vi "Data Viewer.vi"(8 "error in (no error)":errorcluster, 10 "Starting Waveforms":waveform(dbl)[](array[waveform])) -> (0 "error out":errorcluster, 3 "Data Viewer out":refnum<class "Task Viewer.lvclass">)   [LabVIEW 2020, in "Task Viewer.lvlib" / "Task Viewer.lvclass"]
doc: "Initializes the Data Viewer Panel Actor.\n----\nCopyright: MGI 2017\nAuthor: Derek Trepanier"
uses:
  Task Viewer.lvclass
  Task Viewer.lvclass/Task Viewer.ctl
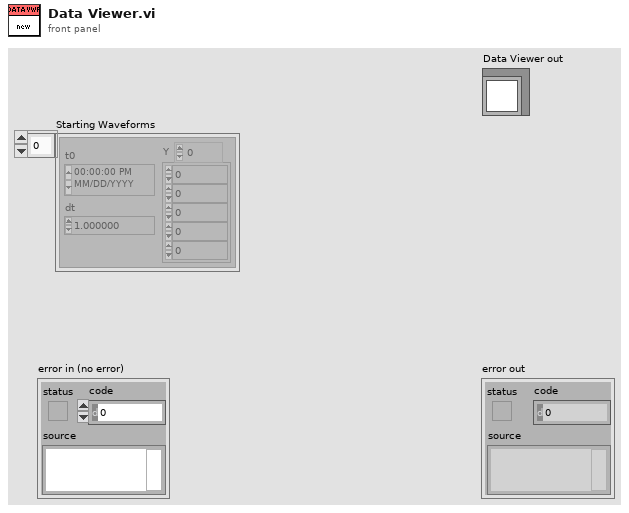
[diagram p1: front panel]
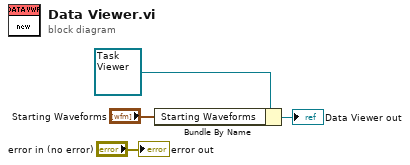
[diagram p0: block diagram]
diagram:
  n1 = Bundle By Name(cluster=refnum<class "Task Viewer.lvclass"> refnum ("Data Viewer in"), "Starting Waveforms"="Starting Waveforms") -> (→"Data Viewer out":refnum<class "Task Viewer.lvclass">)
  "error out" <- "error in (no error)"
